vi "WPI_ADI_IMU_KalmanPitchRollCalcs.vi"(0 "Accel":dbl, 1 "Gyro":dbl, 2 "dt (ms)":dbl, 3 "Q_Angle":dbl=0.001 format="%#_13g", 4 "Q_Bias":dbl=0.001 format="%#_13g", 5 "R_Measure":dbl=0.01 format="%#_13g") -> (14 "Filtered":dbl)   [LabVIEW 2015]
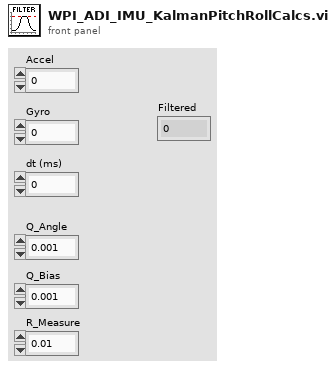
[diagram p1: front panel]
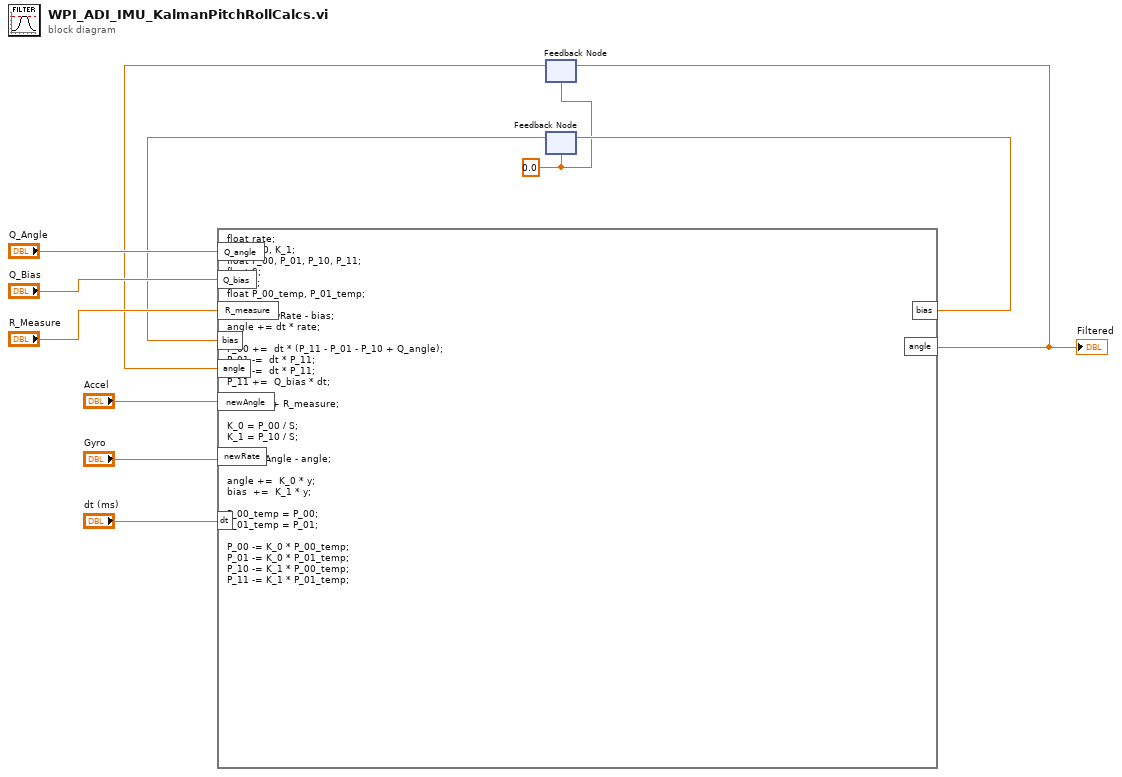
[diagram p0: block diagram]
diagram:
  w5 = 0.0 ("x_bias")
  n1 = feedback #1(w5) -> (w2:dbl)
  n2 = feedback #2(w5) -> (w3:dbl)
  n3 = formula code="float rate;\nfloat K_0, K_1;\nfloat P_00, P_01, P_10, P_11;\nfloat S;\nfloat y;\nfloat P_00_temp, P_01_temp;\n\nrate = newRate - bias;\nangle += dt * rate;\n\nP_00 +=  dt * (P_11 - P_01 - P_10 + Q_angle);\nP_01 -=  dt * P_11;\nP_10 -=  dt * P_11;\nP_11 +=  Q_bias * dt;\n\nS = P_00 + R_measure;\n\nK_0 = P_00 / S;\nK_1 = P_10 / S;\n\ny = newAngle - angle;\n\nangle +=  K_0 * y;\nbias  +=  K_1 * y;\n\nP_00_temp = P_00;\nP_01_temp = P_01;\n\nP_00 -= K_0 * P_00_temp;\nP_01 -= K_0 * P_01_temp;\nP_10 -= K_1 * P_00_temp;\nP_11 -= K_1 * P_01_temp;"("dt"="dt (ms)", "Q_angle"="Q_Angle", "Q_bias"="Q_Bias", "R_measure"="R_Measure", "bias"=w3, "newAngle"="Accel", "newRate"="Gyro", "angle"=w2) -> ("angle"=w4:dbl, "bias"=w8:dbl)
  "Filtered" <- w4
  n4 = feedback-in #1(w4) -> ()
  n5 = feedback-in #2(w8) -> ()
